vi "Hysteresis.vi"(5 "level":dbl format="%.2p", 7 "hysteresis":dbl format="%.2p", 9 "signal in":waveform(dbl), 11 "error in (no error)":errorcluster) -> (8 "ACT_Dv_too_large":bool, 15 "error out":errorcluster)   [LabVIEW 2022 SP3]
uses:
  <vilib>/measure/mamon.llb/Trigger Detection for 1 Channel.vi
  <vilib>/measure/NI_MAPro.lvlib
panel:
  in  "location mode":u16(ring) items=["Index", "Time"]
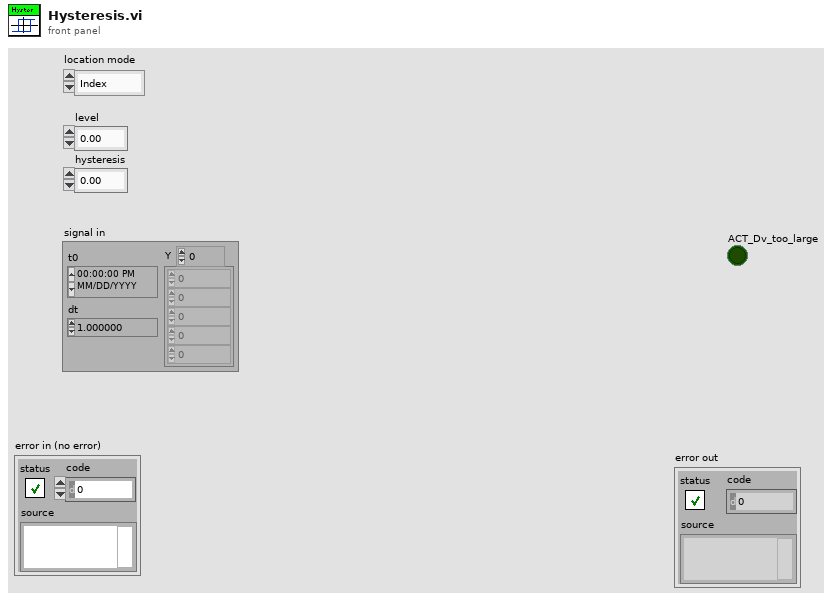
[diagram p1: front panel]
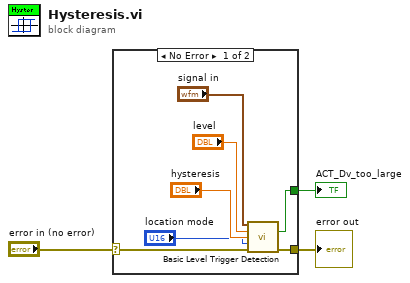
[diagram p0: block diagram]
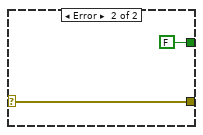
[diagram p2: hidden frame]
diagram:
  n1 = case shown="No Error" "error in (no error)" {
    selector: "error in (no error)" -> [w9 w12]
    tunnel: [w8 w12] -> w2
    tunnel: [w4 FALSE ("trigger detected?")] -> w1
    frame No Error {
      n2 = call-poly <vilib>:"Basic Level Trigger Detection.vi"("signal in"="signal in", "level"="level", "hysteresis"="hysteresis", "location mode"="location mode", "error in (no error)"=w9) -> ("trigger detected?"=w4:bool, "error out"=w8:errorcluster)  [unwired: 8 in, 1 out]
    }
    frame Error {
    }
  }
  "error out" <- w2
  "ACT_Dv_too_large" <- w1
